vi "AudioEqualizer.vi"() -> ()   [LabVIEW 2021]
uses:
  <vilib>/express/express analysis/Spectral/Block/exnSpectralBlock spectral measurements power poly.vi
  <vilib>/express/express analysis/Spectral/Block/exnSpectralBlock spectral measurements power DDT.vi
  <vilib>/express/express analysis/Spectral/XNode/ExpressSpectralMeasurementsBlockNode.xnode
panel:
  in  "Treble":dbl(slide) scale=0.0..1.0
  in  "Midrange":dbl(slide) scale=0.0..1.0
  in  "Bass":dbl(slide) scale=0.0..1.0
  in  "Volume":dbl(slide) scale=0.0..1.0
  out "AUX OUT":dynamicdata(graph)
  out "AUX IN":dynamicdata(graph)
  in  "stop":bool
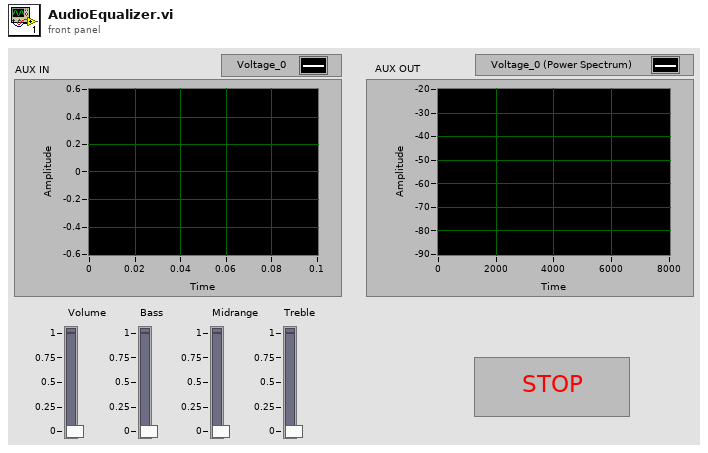
[diagram p1: front panel]
types:
  T1 = cluster{"averaging mode":u16, "weighting mode":u16, "number of averages":u32}
  T2 = cluster{"dB On (F)":bool, "unwrap phase (F)":bool, "convert to degree (F)":bool}
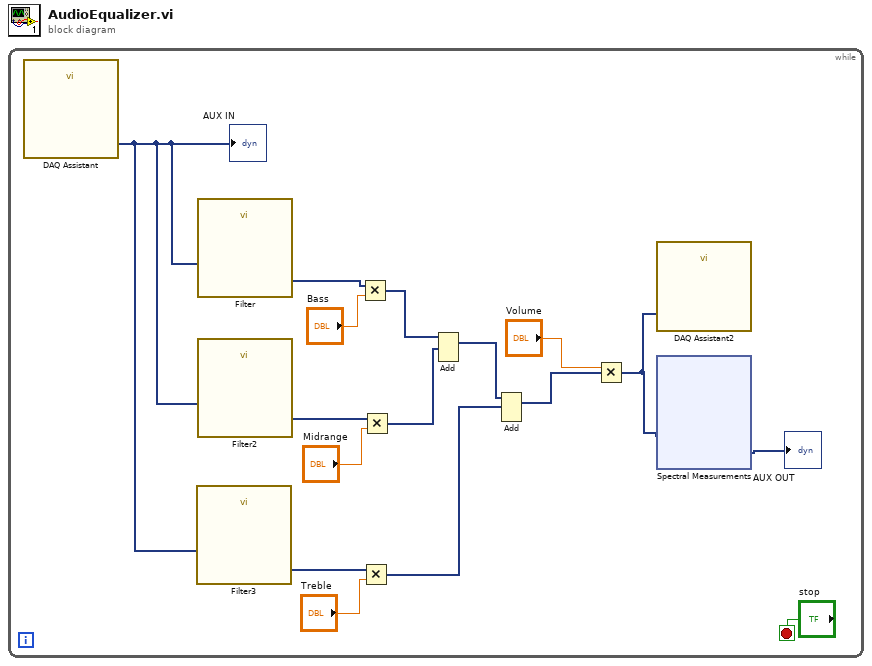
[diagram p0: block diagram]
diagram:
  n1 = while {
    stop <- "stop" stop-if-true
    n2 = call "DAQ Assistant"() -> ("data"=w6:dynamicdata)  [unwired: 16 in, 3 out]
    "AUX IN" <- w6
    n3 = call "Filter3"("Signal"=w6) -> ("Filtered Signal"=w5:dynamicdata)  [unwired: 9 in, 1 out]
    n4 = call "Filter"("Signal"=w6) -> ("Filtered Signal"=w3:dynamicdata)  [unwired: 9 in, 1 out]
    n5 = call "Filter2"("Signal"=w6) -> ("Filtered Signal"=w4:dynamicdata)  [unwired: 9 in, 1 out]
    n6 = Multiply(x=w3, y="Bass") -> (x*y=w12:dynamicdata)
    n7 = Multiply(x=w5, y="Treble") -> (x*y=w10:dynamicdata)
    n8 = Multiply(x=w4, y="Midrange") -> (x*y=w11:dynamicdata)
    n9 = Add(1:w11, 2:w12) -> (0:w9:dynamicdata)  [unwired: 1 in, 1 out]
    n10 = Add(1:w10, 2:w9) -> (0:w8:dynamicdata)  [unwired: 1 in, 1 out]
    n11 = Multiply(x="Volume", y=w8) -> (x*y=w1:dynamicdata)
    n12 = call "DAQ Assistant2"("data"=w1) -> ()  [unwired: 16 in, 3 out]
    n13 = xnode "Spectral Measurements"("Signals"=w1) -> ("Power Spectrum"=→"AUX OUT":dynamicdata)  [unwired: 1 in, 1 out]
  }
